vi "ZMC Get Errcode Description.vi"(8 "error in (no error)":errorcluster caption="错误输入（无错误）", 11 "ierrcode":i32) -> (0 "error out":errorcluster caption="错误输出", 3 "function return":string)   [LabVIEW 2015, in "zauxdll.lvlib"]
doc: "const char* ZMC_GetErrcodeDescription(int32 ierrcode);"
uses:
  zauxdll.lvlib
  zmotion.dll
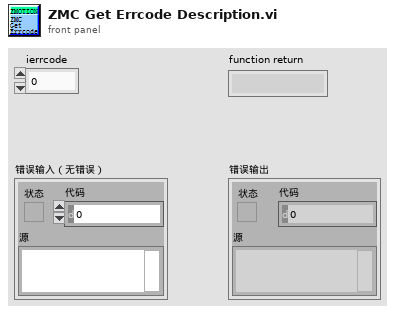
[diagram p1: front panel]
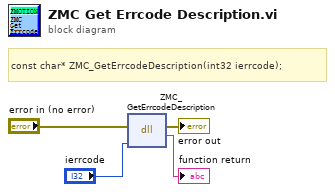
[diagram p0: block diagram]
diagram:
  # "const char* ZMC_GetErrcodeDescription(int32 ierrcode);"
  n1 = dll-call lib="C:/Users/VIC/Desktop/GOGORO_SA/system/LLB/zmotion/zaux/zmotion.*" fn="ZMC_GetErrcodeDescription"(error in="error in (no error)", "ierrcode"="ierrcode") -> (error out=→"error out":errorcluster, →"function return":string)  [unwired: 3 in, 1 out]
